vi "CameraTool Class Sandbox.vi"() -> ()   [LabVIEW 2011]
uses:
  CameraTool Class.lvclass
panel:
  out "error out":errorcluster
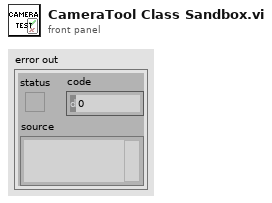
[diagram p1: front panel]
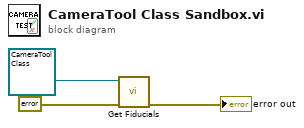
[diagram p0: block diagram]
diagram:
  n1 = call "Get Fiducials.vi"("error in"=errorcluster {"status"=FALSE, "code"=0, "source"=""} ("error constant"), "CameraTool In"=refnum<class "CameraTool Class.lvclass"> refnum ("CameraTool Class in")) -> ("error out"=→"error out":errorcluster)  [unwired: 4 in, 3 out]
